vi "Localize This VI.vi"   [LabVIEW 2017]
uses:
  API/JKI Simple Localization.lvlib
types:
  T1 = enum32{"invalid OS target", "Mac OS", "Windows 3.1", "Windows 95/NT", "Solaris 1", "Solaris 2", "HP-UX", "PowerMAX", "Linux", "Irix", "Rhapsody", "BeOS", "AIX", "OSF1", "VxWorks", "PharLap", "Carbon", "RTX", "Windows x64", "Linux x64", "Mac OS X x64"}
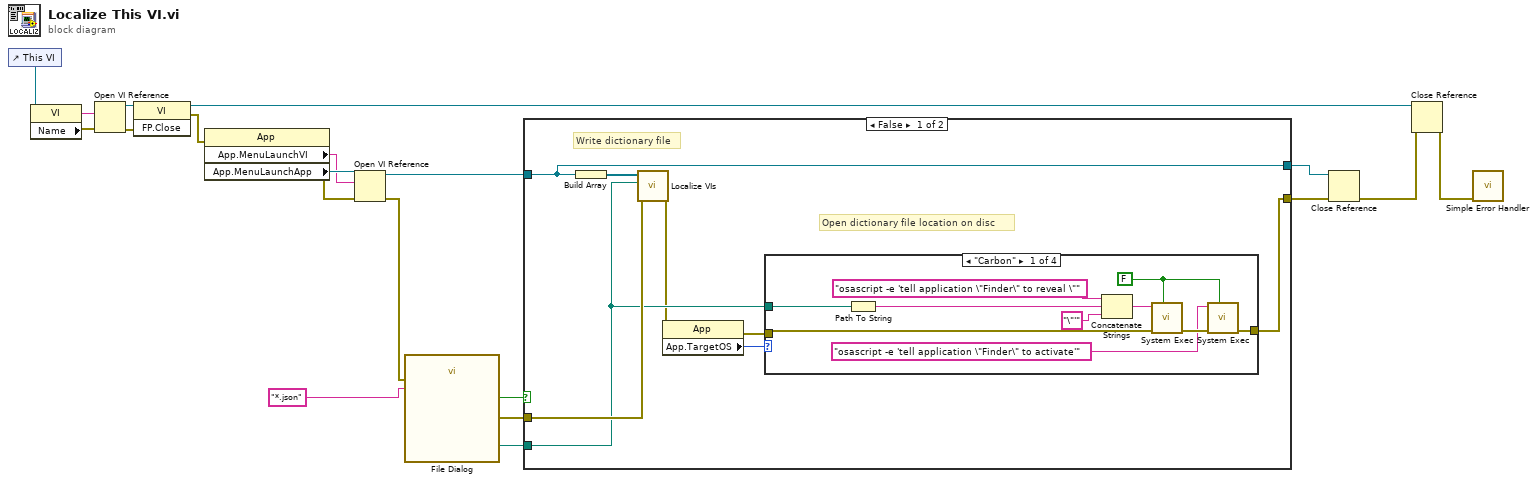
[diagram p0: block diagram]
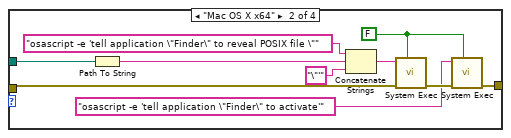
[diagram p2: hidden frame]
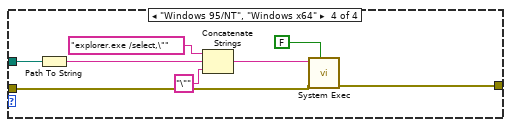
[diagram p4: hidden frame]
diagram:
  n1 = control-ref of="This VI"() -> (w16:refnum<vi>)
  n2 = property class="VI"(reference=w16) -> (error out=w12:errorcluster, "Name"=w15:string)  [unwired: 1 in, 1 out]
  n3 = Open VI Reference(vi path=w15, error in (no error)=w12) -> (vi reference=w14:refnum<vi>, error out=w11:errorcluster)  [unwired: 4 in]
  n4 = invoke class="VI" method="FP.Close"(reference=w14, error in=w11) -> (reference out=w10:refnum<vi>, error out=w13:errorcluster)  [unwired: 1 in, 1 out]
  n5 = property class="App"(error in=w13) -> (error out=w18:errorcluster, "App.MenuLaunchVI"=w19:string, "App.MenuLaunchApp"=w20:refnum<vi>)  [unwired: 1 in, 1 out]
  n6 = Open VI Reference(application reference (local)=w20, vi path=w19, error in (no error)=w18) -> (vi reference=w8:refnum<vi>, error out=w17:errorcluster)  [unwired: 3 in]
  n7 = call "File Dialog"("error in"=w17, "pattern (all files)"="*.json" ("pattern label")) -> ("selected path"=w6:path, "cancelled"=w4:bool, "error out"=w5:errorcluster)  [unwired: 10 in, 1 out]
  n8 = case shown="False" w4 {
    tunnel: w8 -> [w26 w59]
    tunnel: w6 -> [w24 _]
    tunnel: w5 -> [w27 w58]
    tunnel: [w26 w59] -> w3
    tunnel: [w21 w58] -> w2
    frame False {
      # "Open dictionary file location on disc"
      # "Write dictionary file"
      n9 = Build Array(w26) -> (w28:refnum<vi>[])
      n10 = call "Localize VIs.vi"("error in (no error)"=w27, "Dictionary Path"=w24, "VIs in"=w28) -> ("error out"=w23:errorcluster)  [unwired: 8 in]
      n11 = property class="App"(error in=w23) -> (error out=w22:errorcluster, "App.TargetOS"=w25:T1)  [unwired: 1 in, 1 out]
      n12 = case shown="\"Carbon\"" w25 {
        tunnel: w24 -> [w31 w43 _ w53]
        tunnel: w22 -> [w29 w39 w49 w51]
        tunnel: [w30 w40 w49 w50] -> w21
        frame "Carbon" {
          w34 = FALSE ("wait until completion? (T)")
          n13 = Path To String(path=w31) -> (string=w32:string)
          n14 = Concatenate Strings("osascript -e 'tell application \"Finder\" to reveal \"" ("string"), w32, "\"'" ("string")) -> (w36:string)
          n15 = call <vilib>:"System Exec.vi"("wait until completion? (T)"=w34, "error in (no error)"=w29, "command line"=w36) -> ("error out"=w35:errorcluster)  [unwired: 5 in, 3 out]
          n16 = call <vilib>:"System Exec.vi"("wait until completion? (T)"=w34, "error in (no error)"=w35, "command line"="osascript -e 'tell application \"Finder\" to activate'" ("string")) -> ("error out"=w30:errorcluster)  [unwired: 5 in, 3 out]
        }
        frame "Mac OS X x64" {
          w45 = FALSE ("wait until completion? (T)")
          n17 = Path To String(path=w43) -> (string=w42:string)
          n18 = Concatenate Strings("osascript -e 'tell application \"Finder\" to reveal POSIX file \"" ("string"), w42, "\"'" ("string")) -> (w47:string)
          n19 = call <vilib>:"System Exec.vi"("wait until completion? (T)"=w45, "error in (no error)"=w39, "command line"=w47) -> ("error out"=w46:errorcluster)  [unwired: 5 in, 3 out]
          n20 = call <vilib>:"System Exec.vi"("wait until completion? (T)"=w45, "error in (no error)"=w46, "command line"="osascript -e 'tell application \"Finder\" to activate'" ("string")) -> ("error out"=w40:errorcluster)  [unwired: 5 in, 3 out]
        }
        frame Default {
        }
        frame "Windows 95/NT", "Windows x64" {
          n21 = Path To String(path=w53) -> (string=w52:string)
          n22 = Concatenate Strings("explorer.exe /select,\"" ("string"), w52, "\"" ("string")) -> (w55:string)
          n23 = call <vilib>:"System Exec.vi"("wait until completion? (T)"=FALSE, "error in (no error)"=w51, "command line"=w55) -> ("error out"=w50:errorcluster)  [unwired: 5 in, 3 out]
        }
      }
    }
    frame True {
    }
  }
  n24 = Close Reference(reference=w3, error in (no error)=w2) -> (error out=w7:errorcluster)
  n25 = Close Reference(reference=w10, error in (no error)=w7) -> (error out=w9:errorcluster)
  n26 = call <vilib>:"Simple Error Handler.vi"("error in (no error)"=w9) -> ()  [unwired: 4 in, 5 out]
